vi "vec2.vi"(7 "scale (1/x)":dbl=1.0, 8 "y":dbl, 10 "x":dbl) -> (2 "Vec2":T1)   [LabVIEW 2020]
uses:
  vec2.ctl
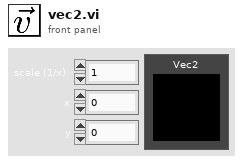
[diagram p1: front panel]
types:
  T1 = typedef "vec2.ctl" = cluster{"X":dbl, "Y":dbl}[]
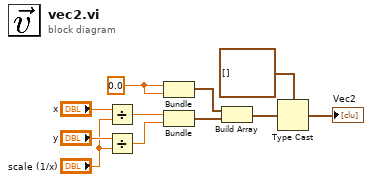
[diagram p0: block diagram]
diagram:
  w11 = 0.0 ("x")
  n1 = Divide(x="x", y="scale (1/x)") -> (x/y=w2:dbl)
  n2 = Divide(x="y", y="scale (1/x)") -> (x/y=w1:dbl)
  n3 = Bundle("x"=w11, "x"=w11) -> (w10:cluster{"x":dbl, "x":dbl})  [unwired: 1 in]
  n4 = Bundle(w2, w1) -> (w9:cluster{dbl, dbl})  [unwired: 1 in]
  n5 = Build Array(w10, w9) -> (w7:cluster{"x":dbl, "x":dbl}[])
  n6 = Type Cast(type=T1 [] ("Vec2"), x=w7) -> (*(type *) &x=→"Vec2":T1)
